vi "Prompt Operator during Motion.vi"(8 "error in (no error)":errorcluster, 11 "Sequence in":refnum<class "Sequence.lvclass">) -> (0 "error out":errorcluster, 1 "Prompt Operator RF In/Out":bool, 3 "Sequence out":refnum<class "Sequence.lvclass">)   [LabVIEW 2018, in "Sequence.lvclass"]
doc: "Contain the user prompt logic in a subvi, applies to motion mode only.\nIn the motion configuration, the operator will still need to manually connect the PNA to the board RF IN and RF OUT ports during fully automated testing. This VI determines when to prompt the operator to re-patch.\nThis indicator is ignored when not in motion mode"
uses:
  Sequence.lvclass
  Sequence.lvclass/Sequence.ctl
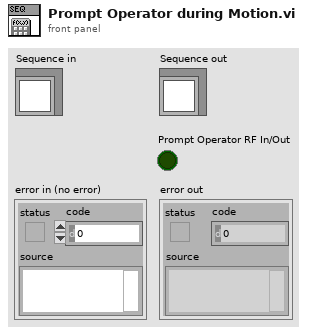
[diagram p1: front panel]
types:
  T1 = typedef "RF Direction.ctl" = enum16{"Tx - RF In", "Rx - RF Out"}
  T2 = typedef "mWaveTestStep.ctl" = cluster{"StepType":T3, "RF In/Out":T1, "Module/Raster":i32, "Polarization":T4, "AO-64 Array":dbl[], "Position":T5[]}
  T3 = typedef "TestStepTypes.ctl" = enum16{"MotionFF-M2", "Motion", "SweepTest", "RasterTest", "Finish", "64ModuleCfg"}
  T4 = typedef "PolarizationSelect.ctl" = enum16{"Vertical", "Horizontal"}
  T5 = typedef "singleAxisMoveDef.ctl" = cluster{"mmWave Axis":T6, "eng. value":dbl}
  T6 = typedef "mmWaveAxis.ctl" = string
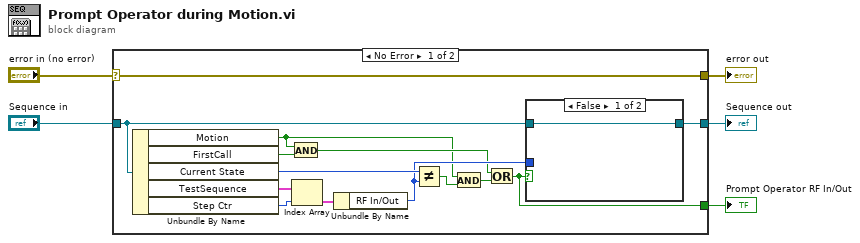
[diagram p0: block diagram]
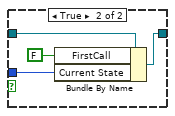
[diagram p2: hidden frame]
diagram:
  n1 = case shown="No Error" "error in (no error)" {
    selector: "error in (no error)" -> [w19 w26]
    tunnel: [w19 w26] -> w4
    tunnel: [w12 w25] -> w2
    tunnel: "Sequence in" -> [w13 w25]
    tunnel: [w6 _] -> w1
    frame No Error {
      n2 = Unbundle By Name(w13) -> ("Motion"=w8:bool, "FirstCall"=w14:bool, "Current State"=w15:T1, "TestSequence"=w17:T2[], "Step Ctr"=w16:i32)
      n3 = And(x=w8, y=w14) -> (x .and. y?=w10:bool)
      n4 = Index Array(array=w17, index=w16) -> (element=w18:T2)
      n5 = Unbundle By Name(w18) -> ("RF In/Out"=w11:T1)
      n6 = Not Equal?(x=w15, y=w11) -> (x != y?=w9:bool)
      n7 = And(x=w8, y=w9) -> (x .and. y?=w7:bool)
      n8 = Or(x=w10, y=w7) -> (x .or. y?=w6:bool)
      n9 = case shown="False" w6 {
        tunnel: w13 -> [w20 w24]
        tunnel: [w20 w23] -> w12
        tunnel: w11 -> [_ w21]
        frame False {
        }
        frame True {
          n10 = Bundle By Name(cluster=w24, "FirstCall"=FALSE ("RF In/Out.FirstCall"), "Current State"=w21) -> (w23:refnum<class "Sequence.lvclass">)
        }
      }
    }
    frame Error {
    }
  }
  "error out" <- w4
  "Sequence out" <- w2
  "Prompt Operator RF In/Out" <- w1
